vi "CSGaussmeter.ProcEvents.vi"(0 "i ref in":refnum<vi>, 5 "error in (no error)":errorcluster) -> (14 "i ref out":refnum<vi>, 19 "error out":errorcluster)   [LabVIEW 2014, in "CSGaussmeter.lvlib"]
doc: "This method is used to define the events the object will listen to. Add your own events here."
uses:
  CSGaussmeter.lvlib
  CSCore/BaseProcess/BaseProcess.event definition.ctl
  CSCore/CAEObj/CAEObj.event definition.ctl
  CSCore/BaseProcess/BaseProcess.descriptor string definition.ctl
  CSCore/BaseProcess/BaseProcess.lvlib
  CSCore/CAEObj/CAEObj.lvlib
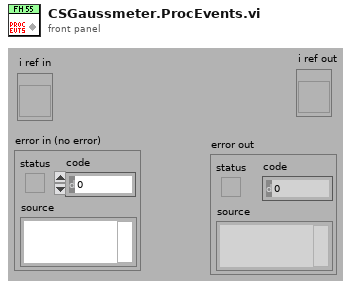
[diagram p1: front panel]
types:
  T1 = typedef "BaseProcess.lvlib/BaseProcess.event definition.ctl" = cluster{"CAEEvtDef":T2, "Data Descriptor":T3}
  T2 = typedef "CAEObj.lvlib/CAEObj.event definition.ctl" = cluster{"URL":string, "enable":bool, "ignoreResID":bool}
  T3 = typedef "BaseProcess.lvlib/BaseProcess.descriptor string definition.ctl" = string
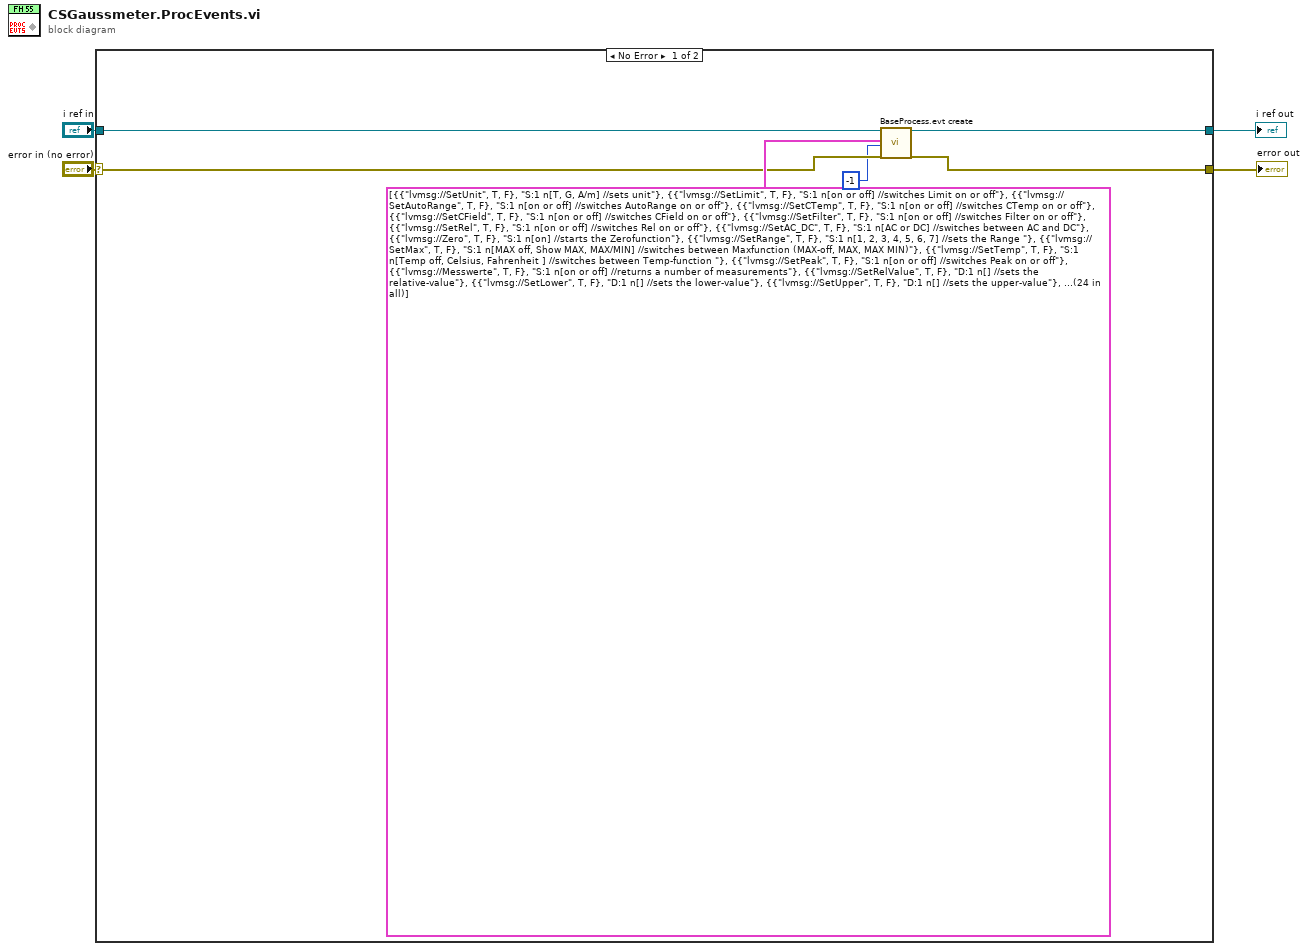
[diagram p0: block diagram]
diagram:
  n1 = case shown="No Error" "error in (no error)" {
    selector: "error in (no error)" -> [w6 w11]
    tunnel: "i ref in" -> [w10 w12]
    tunnel: [w9 w12] -> w3
    tunnel: [w8 w11] -> w2
    frame No Error {
      n2 = call "BaseProcess.evt create.vi"("i ref in"=w10, "newEvents"=T1[] [{"CAEEvtDef"={"URL"="lvmsg://SetUnit", "enable"=TRUE, "ignoreResID"=FALSE}, "Data Descriptor"="S:1 n[T, G, A/m] //sets unit"}, {"CAEEvtDef"={"URL"="lvmsg://SetLimit", "enable"=TRUE, "ignoreResID"=FALSE}, "Data Descriptor"="S:1 n[on or off] //switches Limit on or off"}, {"CAEEvtDef"={"URL"="lvmsg://SetAutoRange", "enable"=TRUE, "ignoreResID"=FALSE}, "Data Descriptor"="S:1 n[on or off] //switches AutoRange on or off"}, {"CAEEvtDef"={"URL"="lvmsg://SetCTemp", "enable"=TRUE, "ignoreResID"=FALSE}, "Data Descriptor"="S:1 n[on or off] //switches CTemp on or off"}, {"CAEEvtDef"={"URL"="lvmsg://SetCField", "enable"=TRUE, "ignoreResID"=FALSE}, "Data Descriptor"="S:1 n[on or off] //switches CField on or off"}, {"CAEEvtDef"={"URL"="lvmsg://SetFilter", "enable"=TRUE, "ignoreResID"=FALSE}, "Data Descriptor"="S:1 n[on or off] //switches Filter on or off"}, {"CAEEvtDef"={"URL"="lvmsg://SetRel", "enable"=TRUE, "ignoreResID"=FALSE}, "Data Descriptor"="S:1 n[on or off] //switches Rel on or off"}, {"CAEEvtDef"={"URL"="lvmsg://SetAC_DC", "enable"=TRUE, "ignoreResID"=FALSE}, "Data Descriptor"="S:1 n[AC or DC] //switches between AC and DC"}, {"CAEEvtDef"={"URL"="lvmsg://Zero", "enable"=TRUE, "ignoreResID"=FALSE}, "Data Descriptor"="S:1 n[on] //starts the Zerofunction"}, {"CAEEvtDef"={"URL"="lvmsg://SetRange", "enable"=TRUE, "ignoreResID"=FALSE}, "Data Descriptor"="S:1 n[1, 2, 3, 4, 5, 6, 7] //sets the Range "}, {"CAEEvtDef"={"URL"="lvmsg://SetMax", "enable"=TRUE, "ignoreResID"=FALSE}, "Data Descriptor"="S:1 n[MAX off, Show MAX, MAX/MIN] //switches between Maxfunction (MAX-off, MAX, MAX MIN)"}, {"CAEEvtDef"={"URL"="lvmsg://SetTemp", "enable"=TRUE, "ignoreResID"=FALSE}, "Data Descriptor"="S:1 n[Temp off, Celsius, Fahrenheit ] //switches between Temp-function "}, {"CAEEvtDef"={"URL"="lvmsg://SetPeak", "enable"=TRUE, "ignoreResID"=FALSE}, "Data Descriptor"="S:1 n[on or off] //switches Peak on or off"}, {"CAEEvtDef"={"URL"="lvmsg://Messwerte", "enable"=TRUE, "ignoreResID"=FALSE}, "Data Descriptor"="S:1 n[on or off] //returns a number of measurements"}, {"CAEEvtDef"={"URL"="lvmsg://SetRelValue", "enable"=TRUE, "ignoreResID"=FALSE}, "Data Descriptor"="D:1 n[] //sets the relative-value"}, {"CAEEvtDef"={"URL"="lvmsg://SetLower", "enable"=TRUE, "ignoreResID"=FALSE}, "Data Descriptor"="D:1 n[] //sets the lower-value"}, {"CAEEvtDef"={"URL"="lvmsg://SetUpper", "enable"=TRUE, "ignoreResID"=FALSE}, "Data Descriptor"="D:1 n[] //sets the upper-value"}, {"CAEEvtDef"={"URL"="lvmsg://Reset", "enable"=TRUE, "ignoreResID"=FALSE}, "Data Descriptor"="S:1 n[on] //sets MAX/MIN or Peak values to Zero "}, {"CAEEvtDef"={"URL"="lvmsg://SetLocal", "enable"=TRUE, "ignoreResID"=FALSE}, "Data Descriptor"="S:1 n[on] //turned off the remote control\n"}, {"CAEEvtDef"={"URL"="lvmsg://OK", "enable"=TRUE, "ignoreResID"=FALSE}, "Data Descriptor"="S:1 n[on] //clears the error message"}, {"CAEEvtDef"={"URL"="lvmsg://Init", "enable"=TRUE, "ignoreResID"=FALSE}, "Data Descriptor"="S:1 n[on] //reads all values from the device"}, {"CAEEvtDef"={"URL"="lvmsg://SaveSettings", "enable"=TRUE, "ignoreResID"=FALSE}, "Data Descriptor"="C:N n[on] //reads all values from the device"}, {"CAEEvtDef"={"URL"="lvmsg://LoadSettings", "enable"=TRUE, "ignoreResID"=FALSE}, "Data Descriptor"="C:N n[on] //reads all values from the device"}, {"CAEEvtDef"={"URL"="lvmsg://OpenGUI", "enable"=TRUE, "ignoreResID"=FALSE}, "Data Descriptor"="S:1 n[on] //clears the error message"}] ("new events"), "ms timeout (10000)"=-1, "error in (no error)"=w6) -> ("i ref out"=w9:refnum<vi>, "error out"=w8:errorcluster)  [unwired: 12 in, 2 out]
    }
    frame Error {
    }
  }
  "i ref out" <- w3
  "error out" <- w2
